vi "identColor2.vi"(7 "Parâmetros Ini":T2={"Gyro Port"=0, "Sensor - Left"=3, "Sensor - Right"=2, "     Color \nSensor Port"=1, "Kp Front"=0.5, "Motor speed"=-15, "Distance to street"=0.0, "Motor speed turns"=16, "Kp Curvas"=0.0} {"Kp Front" format="%.3f"; "Color \nSensor Port" items=["Port 1", "Port 2", "Port 3", "Port 4"]; "Sensor - Right" items=["Port 1", "Port 2", "Port 3", "Port 4"]; "Sensor - Left" items=["Port 1", "Port 2", "Port 3", "Port 4"]; "Gyro Port" items=["Port 1", "Port 2", "Port 3", "Port 4"]}, 11 "NXT/EV3":T1) -> (1 "Collor":T4, 3 "NXT/EV3 2":T1)   [LabVIEW 2016]
uses:
  <vilib>/NXT/Subs/LVHSConnector.ctl
  <vilib>/NXT/LegoClasses/BrickReference/BrickReference.lvclass
  <vilib>/NXT/Subs/ColorSensorColors.ctl
  parametros.ctl
  <vilib>/NXT/Block Support/NXT_InputPort.ctl
  <vilib>/NXT/Dual Mode Library/Display/drawText_Center.vi
panel:
  out "Detected Color":T4
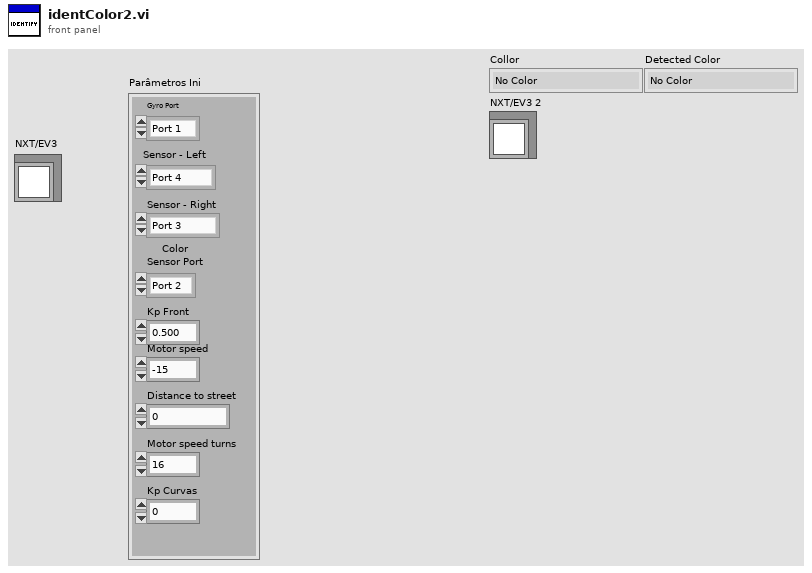
[diagram p1: front panel]
types:
  T1 = typedef "LVHSConnector.ctl" = refnum<class "BrickReference.lvclass">
  T2 = typedef "parametros.ctl" = cluster{"Gyro Port":T3, "Sensor - Left":T3, "Sensor - Right":T3, "     Color \nSensor Port":T3, "Kp Front":dbl, "Motor speed":i32, "Distance to street":dbl, "Motor speed turns":i32, "Kp Curvas":dbl}
  T3 = typedef "NXT_InputPort.ctl" = u32
  T4 = typedef "ColorSensorColors.ctl" = enum16{"No Color", "Black", "Blue", "Green", "Yellow", "Red", "White", "Brown"}
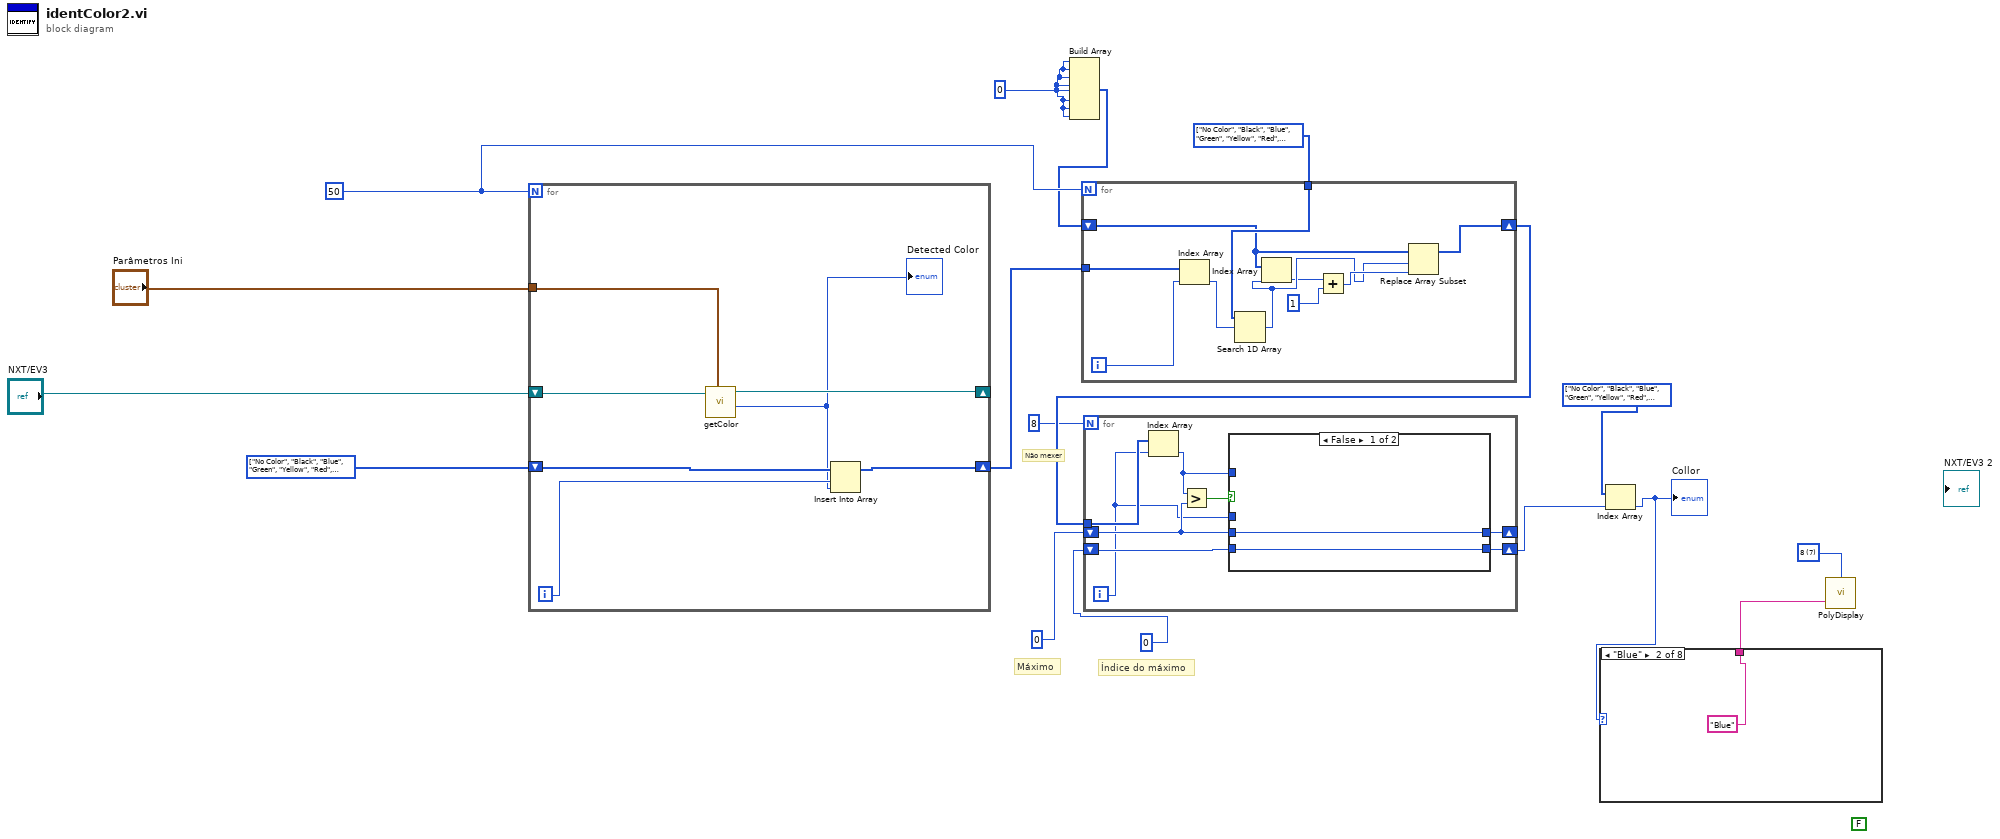
[diagram p0: block diagram]
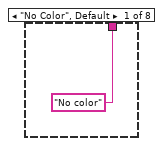
[diagram p2: hidden frame]
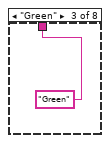
[diagram p3: hidden frame]
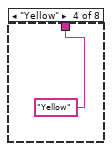
[diagram p4: hidden frame]
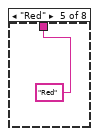
[diagram p5: hidden frame]
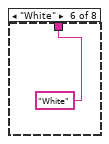
[diagram p6: hidden frame]
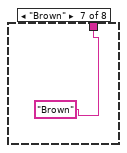
[diagram p7: hidden frame]
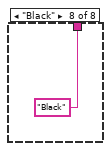
[diagram p8: hidden frame]
diagram:
  (unwired) FALSE
  w3 = i16 7 items=["1", "2", "3", "4", "5", "6", "7", "8", "9", "10", "11", "12"] ("Line")
  w6 = 0
  w7 = T4[] [enum."No Color", enum."Black", enum."Blue", enum."Green", enum."Yellow", enum."Red", enum."White", enum."Brown"] items=["No Color", "Black", "Blue", "Green", "Yellow", "Red", "White", "Brown"]
  w8 = T4[] [enum."No Color", enum."Black", enum."Blue", enum."Green", enum."Yellow", enum."Red", enum."White", enum."Brown"] items=["No Color", "Black", "Blue", "Green", "Yellow", "Red", "White", "Brown"]
  w14 = 50
  w16 = T4[] [enum."No Color", enum."Black", enum."Blue", enum."Green", enum."Yellow", enum."Red", enum."White", enum."Blue"] items=["No Color", "Black", "Blue", "Green", "Yellow", "Red", "White", "Brown"]
  # "Não mexer"
  # "Índice do máximo"
  # "Máximo"
  n1 = for {
    N: w14 -> [_]
    shift-right: [w20] -> _
    shift-left: "NXT/EV3" -> [w21]
    shift-right: [w22] -> w15
    shift-left: w7 -> [w23]
    tunnel: "Parâmetros Ini" -> [w18]
    i -> [w24]
    n2 = call "getColor.vi"("Parâmetros Ini"=w18, "NXT/EV3"=w21) -> ("Cor"=w19:T4, "NXT/EV3 2"=w20:T1)  [unwired: 8 in]
    "Detected Color" <- w19
    n3 = Insert Into Array(array=w23, index=w24, new element=w19) -> (w22:T4[])
  }
  n4 = Build Array(w6, w6, w6, w6, w6, w6, w6, w6) -> (w5:i32[])
  n5 = for {
    N: w14 -> [_]
    tunnel: w15 -> [w33]
    shift-right: [w30] -> w13
    shift-left: w5 -> [w26]
    tunnel: w8 -> [w28]
    i -> [w34]
    n6 = Index Array(array=w33, index=w34) -> (element=w29:T4)
    n7 = Search 1D Array(1D array=w28, element=w29) -> (index of element=w27:i32)  [unwired: 1 in]
    n8 = Index Array(array=w26, index=w27) -> (element=w25:i32)
    n9 = Add(x=w25, y=1) -> (x+y=w31:i32)
    n10 = Replace Array Subset(array=w26, new element=w31, index=w27) -> (w30:i32[])
  }
  n11 = for {
    N: 8 -> [_]
    tunnel: w13 -> [w42]
    shift-right: [w40] -> _
    shift-left: 0 -> [w37]
    shift-right: [w38] -> w9
    shift-left: 0 -> [w36]
    i -> [w35]
    n12 = Index Array(array=w42, index=w35) -> (element=w39:i32)
    n13 = Greater?(x=w39, y=w37) -> (0:w41:bool)
    n14 = case shown="False" w41 {
      tunnel: w37 -> [w44 _]
      tunnel: [w44 w46] -> w40
      tunnel: w39 -> [_ w46]
      tunnel: [w43 w45] -> w38
      tunnel: w36 -> [w43 _]
      tunnel: w35 -> [_ w45]
      frame False {
      }
      frame True {
      }
    }
  }
  n15 = Index Array(array=w16, index=w9) -> (element=w1:T4)
  "Collor" <- w1
  n16 = case shown="\"Blue\"" w1 {
    tunnel: ["No color" "Blue" "Green" "Yellow" "Red" "White" "Brown" "Black"] -> w2
    frame "No Color", Default {
    }
    frame "Blue" {
    }
    frame "Green" {
    }
    frame "Yellow" {
    }
    frame "Red" {
    }
    frame "White" {
    }
    frame "Brown" {
    }
    frame "Black" {
    }
  }
  n17 = call-poly <vilib>:"PolyDisplay.vi"("Text"=w2, "Line"=w3) -> ()  [unwired: 2 in, 1 out]
